vi "ZAlign_FilterControlClass.vi"(0 "SelList[]":refnum<vi>[](array[refnum])) -> (4 "CtrlRefArray":refnum<vi>[](array[refnum]))   [LabVIEW 2014, in "ZAlign.lvlib"]
doc: "ZAlign.lvlib:ZAlign_FilterControlClass.vi\n----------------------------------------------\nSelektierte Controls filtern.\n\nInputs:\n---------------------\n- SelList[] : 1DArrayOfRefnum; \n\nOutputs:\n---------------------\n- CtrlRefArray : 1DArrayOfRefnum; \n\n----------------------------------------------\n26.03.2015 jcm\nZühlke Engineering AG\nCH-8952 Schlieren\nwww.zuehlke.com"
uses:
  ZAlign.lvlib
panel:
  # "Connector Pane"
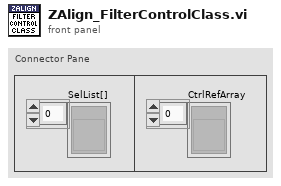
[diagram p1: front panel]
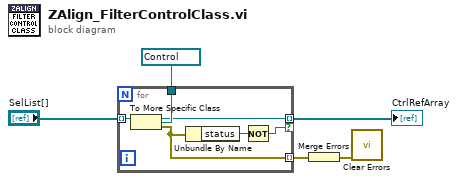
[diagram p0: block diagram]
diagram:
  n1 = for {
    tunnel: refnum<vi> refnum ("reference out") -> [w11]
    tunnel: "SelList[]" -> [w10] mode=indexing
    tunnel: [w9] -> w3 mode=indexing if=w6
    tunnel: [w8] -> w2 mode=indexing
    n2 = To More Specific Class(target class=w11, reference=w10) -> (specific class reference=w9:refnum<vi>, error out=w8:errorcluster)  [unwired: 1 in]
    n3 = Unbundle By Name(w8) -> ("status"=w7:bool)
    n4 = Not(x=w7) -> (.not. x?=w6:bool)
  }
  "CtrlRefArray" <- w3
  n5 = Merge Errors(w2) -> (w1:errorcluster)
  n6 = call <vilib>:"Clear Errors.vi"("error in (no error)"=w1) -> ()  [unwired: 5 in, 2 out]
